vi "AIM664 Timing Control.vi"() -> ()   [LabVIEW 2020]
uses:
  AIM664LV.lvlib
panel:
  out "error out":errorcluster
  out "Irig Out 2":T1
  in  "Irig In 2":T2 {"Control" items=["FDX_IRIG_READ", "FDX_IRIG_WRITE", "FDX_IRIG_EXTERN", "FDX_IRIG_INTERN"]}
  out "Irig Out":T1
  in  "Irig In":T2 {"Control" items=["FDX_IRIG_READ", "FDX_IRIG_WRITE", "FDX_IRIG_EXTERN", "FDX_IRIG_INTERN"]}
  in  "Input Cluster 2":T3={"SrvName"="local", "ClHostName"="local", "ClUser"="Brett", "ClApplication"="Test", "ClApplicationVersion"="V01.00", "ResourceID"=1, "Privileges"=4294967295} {"Privileges" min=4294967295 format="%x"}
  out "NuOfServers":u32=1
  # "ARINC 664 Timing Control"
  # "Overview: This function is used to read or set the on-board IRIG timecode encoder and also to select the IRIG source.  There is a board internal IRIG time source, but it is also possible to synchronize the time coding to an external IRIG source.\n\nRestrictions: None\nInstruction:\n1. Set values \"Set IRIG Time\", change control to FDX_IRIG_WRITE and run the VI\n2. Verify the results in the indicators"
  # "Set Irig Time"
  # "Read Irig Time"
  # "FdxInitCvi"
  # "FdxCmdIrigTimeControlCvi"
  # "FdxLoginCvi"
  # "FdxCmdIrigTimeControlCvi"
  # "FdxLogoutCvi"
  # "Input"
  # "Input"
  # "Output"
  # "Output"
  # "Output"
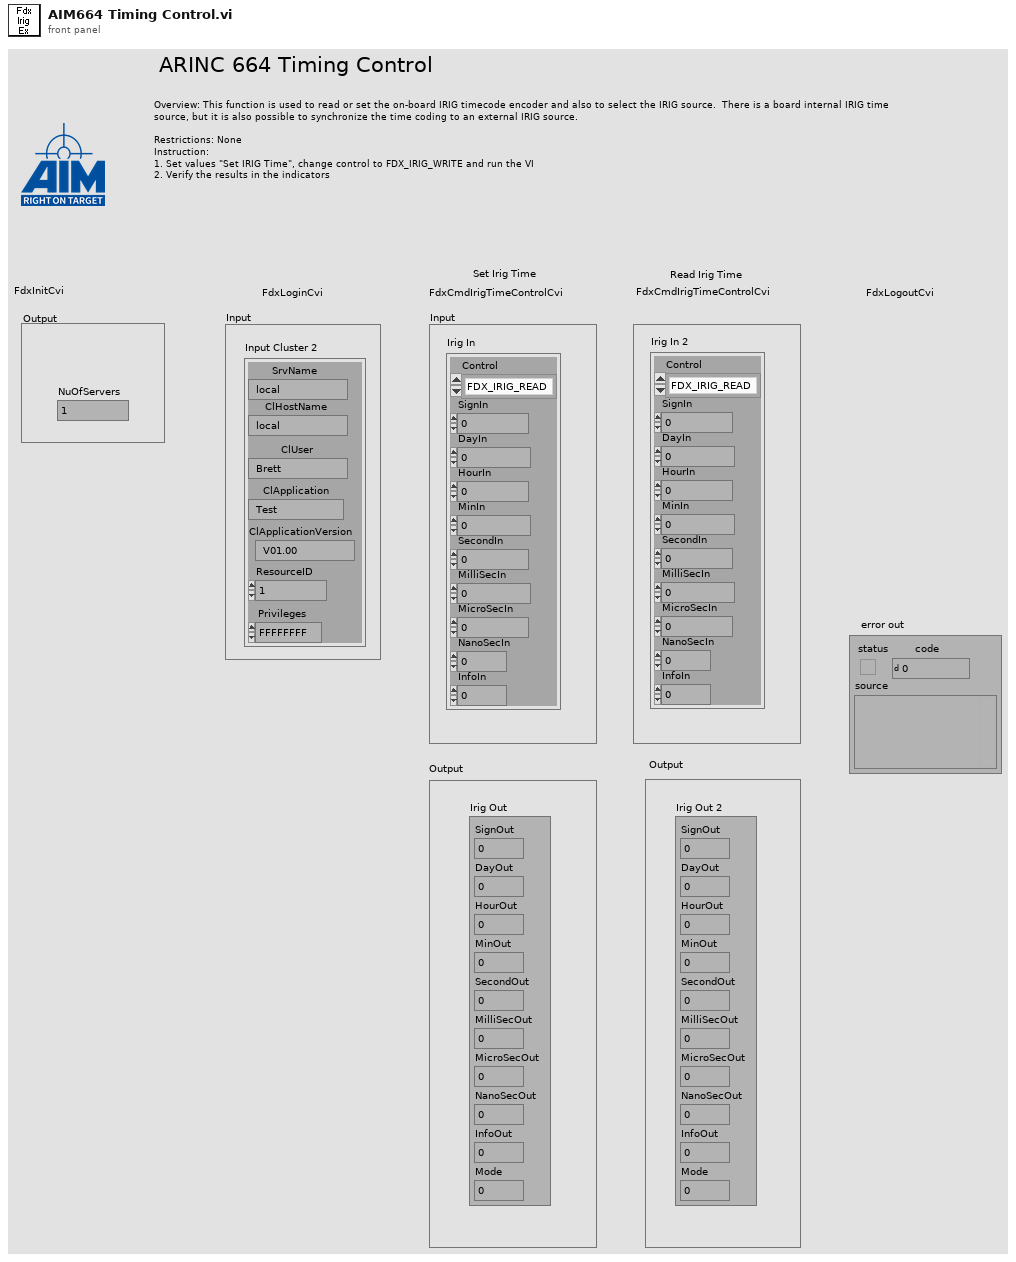
[diagram p1: front panel]
types:
  T1 = cluster{"SignOut":i32, "DayOut":u32, "HourOut":u32, "MinOut":u32, "SecondOut":u32, "MilliSecOut":u32, "MicroSecOut":u32, "NanoSecOut":u32, "InfoOut":u32, "Mode":u32}
  T2 = cluster{"Control":u32, "SignIn":i32, "DayIn":u32, "HourIn":u32, "MinIn":u32, "SecondIn":u32, "MilliSecIn":u32, "MicroSecIn":u32, "NanoSecIn":u32, "InfoIn":u32}
  T3 = cluster{"SrvName":string, "ClHostName":string, "ClUser":string, "ClApplication":string, "ClApplicationVersion":string, "ResourceID":u32, "Privileges":u32}
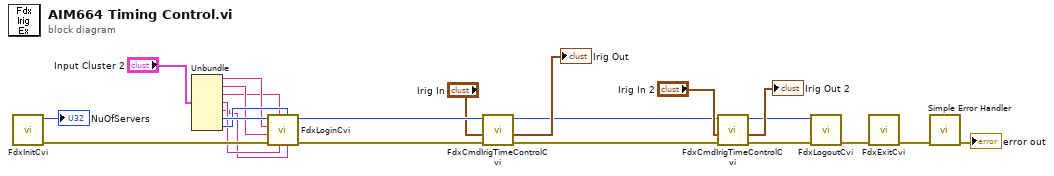
[diagram p0: block diagram]
diagram:
  n1 = call "FdxInitCvi.vi"() -> ("error out"=w22:errorcluster, "Number of Servers"=→"NuOfServers":u32)  [unwired: 10 in]
  n2 = Unbundle("Input Cluster 2") -> ("SrvName"=w7:string, "ClHostName"=w6:string, "ClUser"=w5:string, "ClApplication"=w4:string, "ClApplicationVersion"=w3:string, "ResourceID"=w9:u32, "Privileges"=w8:u32)
  n3 = call "FdxLoginCvi.vi"("ClApplicationVersion"=w3, "Privileges"=w8, "ClApplication"=w4, "ClUser"=w5, "error in"=w22, "ClHostName"=w6, "SrvName"=w7, "ResourceID"=w9) -> ("error out"=w23:errorcluster, "InstrumentHandle"=w18:u32)  [unwired: 2 in]
  n4 = call "FdxCmdIrigTimeControlCvi.vi"("error in"=w23, "Irig In"="Irig In", "InstrumentHandle_board in"=w18) -> ("error out"=w21:errorcluster, "Irig Out"=→"Irig Out":T1, "InstrumentHandle_board out"=w13:u32)  [unwired: 6 in]
  n5 = call "FdxCmdIrigTimeControlCvi.vi"("error in"=w21, "Irig In"="Irig In 2", "InstrumentHandle_board in"=w13) -> ("error out"=w20:errorcluster, "Irig Out"=→"Irig Out 2":T1, "InstrumentHandle_board out"=w12:u32)  [unwired: 6 in]
  n6 = call "FdxLogoutCvi.vi"("error in"=w20, "InstrumentHandle"=w12) -> ("error out"=w19:errorcluster)  [unwired: 9 in]
  n7 = call "FdxExitCvi.vi"("error in"=w19) -> ("error out"=w2:errorcluster)  [unwired: 10 in]
  n8 = call <vilib>:"Simple Error Handler.vi"("error in (no error)"=w2) -> ("error out"=→"error out":errorcluster)  [unwired: 4 in, 4 out]
